vi "SQL_IN Stack Cmd.vi"(11 "parameter buffer":T1) -> (3 "连接的字符串":string)   [LabVIEW 2015]
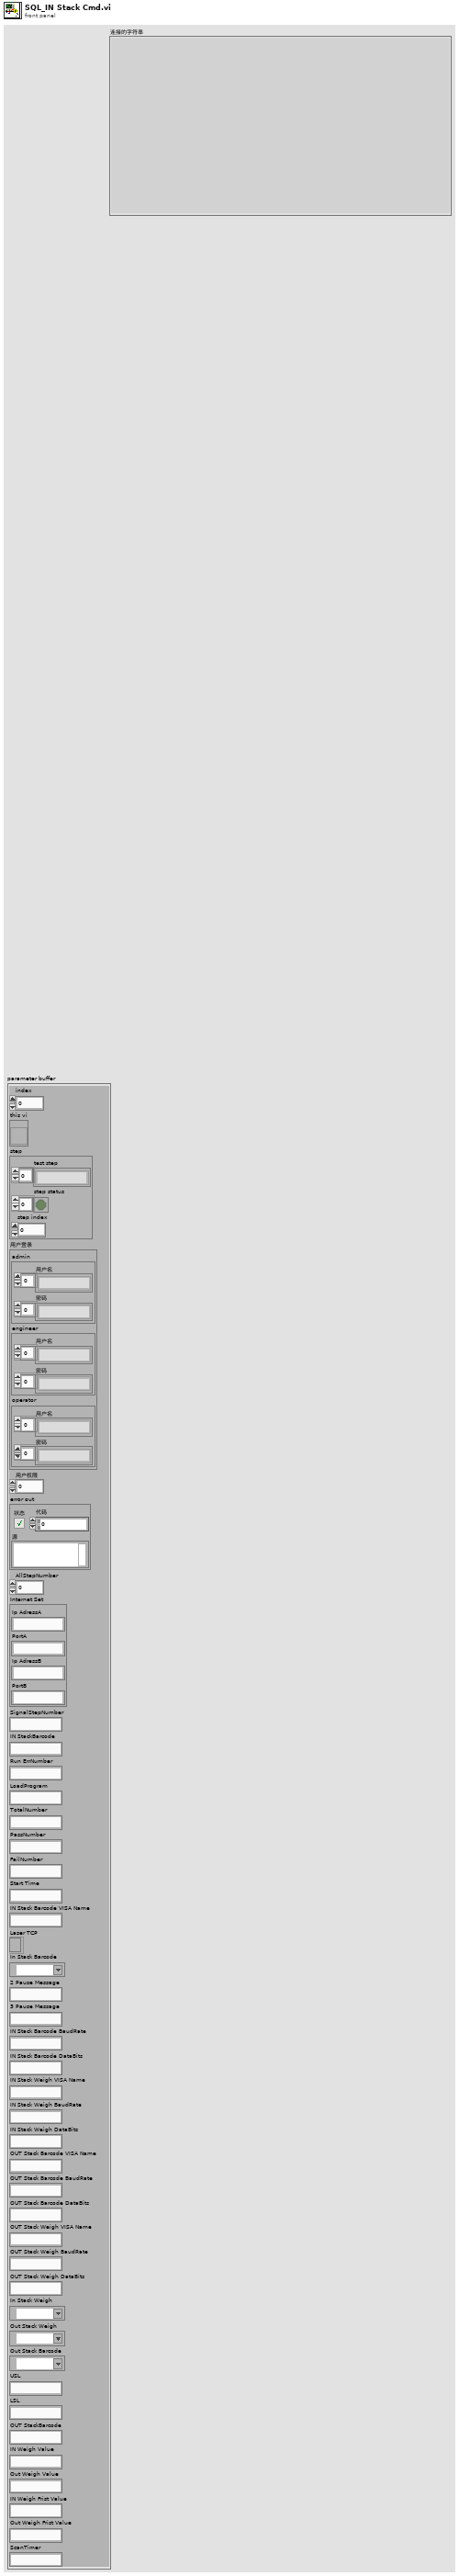
[diagram p1: front panel]
types:
  T1 = cluster{"index":i32, "this vi":refnum<vi>, "step":cluster{"test step":string[], "step status":bool[], "step index":i32}, "用户登录":cluster{"admin":cluster{"用户名":string[], "密码":string[]}, "engineer":cluster{"用户名":string[], "密码":string[]}, "operator":cluster{"用户名":string[], "密码":string[]}}, "用户权限":i32, "error out":errorcluster, "AllStepNumber":i32, "Internet Set":cluster{"Ip AdressA":string, "PortA":string, "Ip AdressB":string, "PortB":string}, "SignalStepNumber":string, "IN StackBarcode":string, "Run ErrNumber":string, "LoadProgram":string, "TotalNumber":string, "PassNumber":string, "FailNumber":string, "Start Time":string, "IN Stack Barcode VISA Name":string, "Laser TCP":refnum<k5>, "In Stack Barcode":refnum<visa-resource-name>, "2 Pause Message":string, "3 Pause Message":string, "IN Stack Barcode BaudRate":string, "IN Stack Barcode DataBits":string, "IN Stack Weigh VISA Name":string, "IN Stack Weigh BaudRate":string, "IN Stack Weigh DataBits":string, "OUT Stack Barcode VISA Name":string, "OUT Stack Barcode BaudRate":string, "OUT Stack Barcode DataBits":string, "OUT Stack Weigh VISA Name":string, "OUT Stack Weigh BaudRate":string, "OUT Stack Weigh DataBits":string, "In Stack Weigh":refnum<visa-resource-name>, "Out Stack Weigh":refnum<visa-resource-name>, "Out Stack Barcode":refnum<visa-resource-name>, "USL":string, "LSL":string, "OUT StackBarcode":string, "IN Weigh Value":string, "Out Weigh Value":string, "IN Weigh Frist Value":string, "Out Weigh Frist Value":string, "ScanTimer":string}
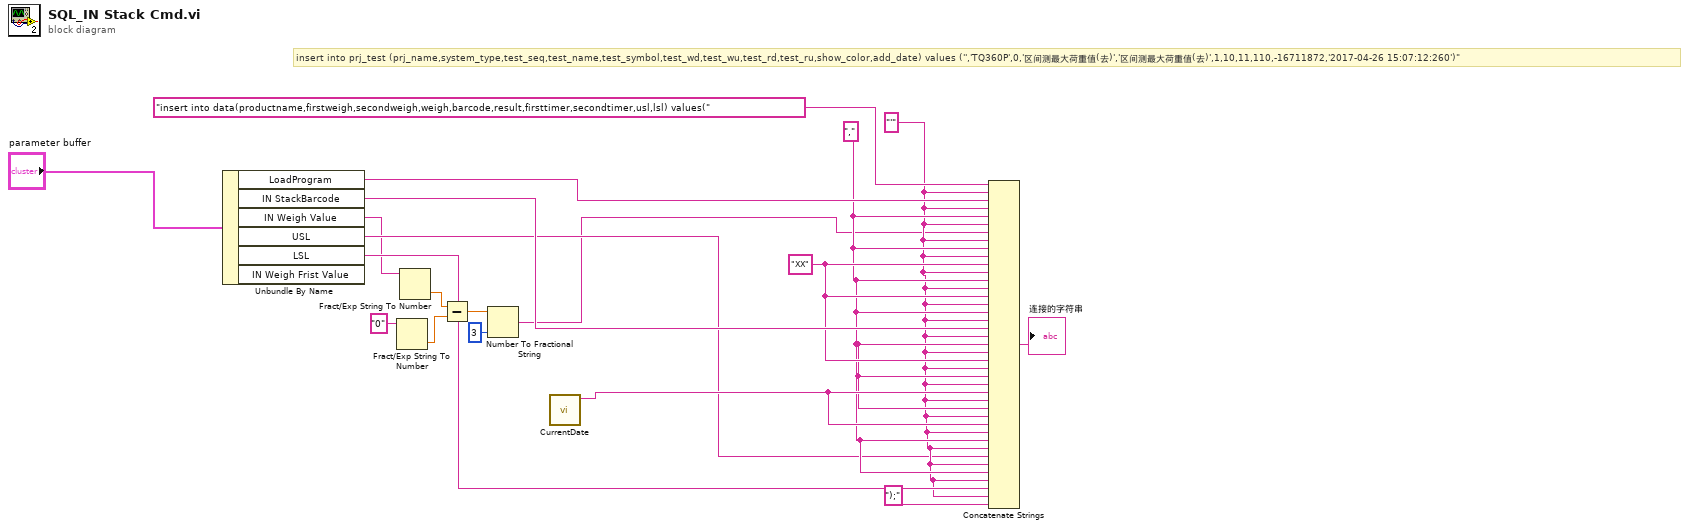
[diagram p0: block diagram]
diagram:
  w16 = "XX" ("字符串")
  w11 = ","
  w10 = "'"
  # "insert into prj_test (prj_name,system_type,test_seq,test_name,test_symbol,test_wd,test_wu,test_rd,test_ru,show_color,add_date) values ('','TQ360P',0,'区间测最大荷重值(去)','区间测最大荷重值(去)',1,10,11,110,-16711872,'2017-04-26 15:07:12:260')\""
  n1 = Unbundle By Name("parameter buffer") -> ("LoadProgram"=w18:string, "IN StackBarcode"=w17:string, "IN Weigh Value"=w4:string, "USL"=w9:string, "LSL"=w14:string)  [unwired: 1 out]
  n2 = Fract/Exp String To Number(string="0" ("字符串")) -> (number=w7:dbl)  [unwired: 3 in, 1 out]
  n3 = Fract/Exp String To Number(string=w4) -> (number=w8:dbl)  [unwired: 3 in, 1 out]
  n4 = Subtract(x=w8, y=w7) -> (x-y=w6:dbl)
  n5 = Number To Fractional String(number=w6, precision (6)=i16 3 ("精度(6)")) -> (F-format string=w3:string)  [unwired: 2 in]
  n6 = call "CurrentDate.vi"() -> ("当前日期时间"=w15:string)  [unwired: 11 in]
  n7 = Concatenate Strings("insert into data(productname,firstweigh,secondweigh,weigh,barcode,result,firsttimer,secondtimer,usl,lsl) values(" ("字符串"), w10, w18, w10, w11, w10, w3, w10, w11, w10, w16, w10, w11, w10, w16, w10, w11, w10, w17, w10, w11, w10, w16, w10, w11, w10, w15, w10, w11, w10, w15, w10, w11, w10, w9, w10, w11, w10, w14, w10, ");") -> (→"连接的字符串":string)
